vi "6-12.vi"() -> ()   [LabVIEW 2017]
uses:
  <vilib>/Utility/file.llb/Read Delimited Spreadsheet (DBL).vi
panel:
  out "Waveform Chart":dbl[](graph)
  out "first row":dbl[](array[numeric])
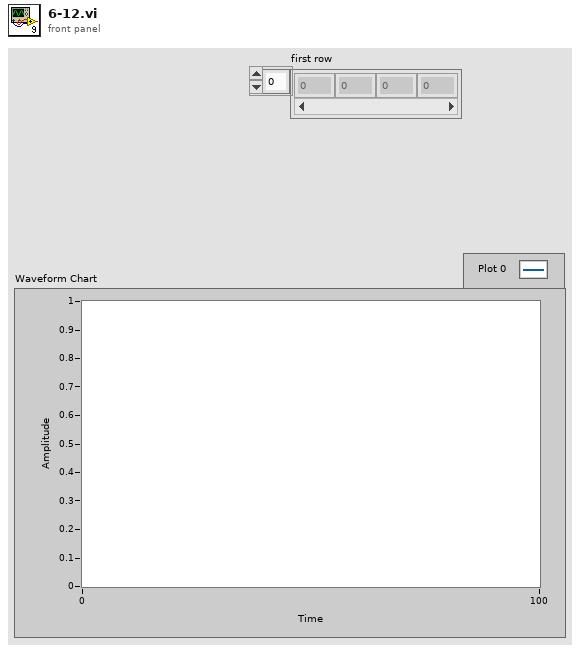
[diagram p1: front panel]
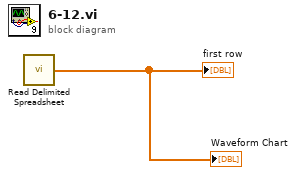
[diagram p0: block diagram]
diagram:
  n1 = call-poly <vilib>:"Read Delimited Spreadsheet.vi"() -> ("first row"=→"first row" →"Waveform Chart":dbl[])  [unwired: 10 in, 5 out]
